vi "sonic info (SubVI).vi"(8 "error in (no error)":errorcluster) -> (0 "error out":errorcluster, 3 "distance to the side":u32)   [LabVIEW 2017]
uses:
  <vilib>/Instr/_visa.llb/VISA Configure Serial Port (Instr).vi
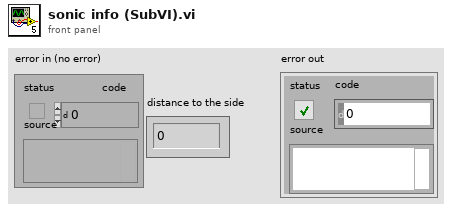
[diagram p1: front panel]
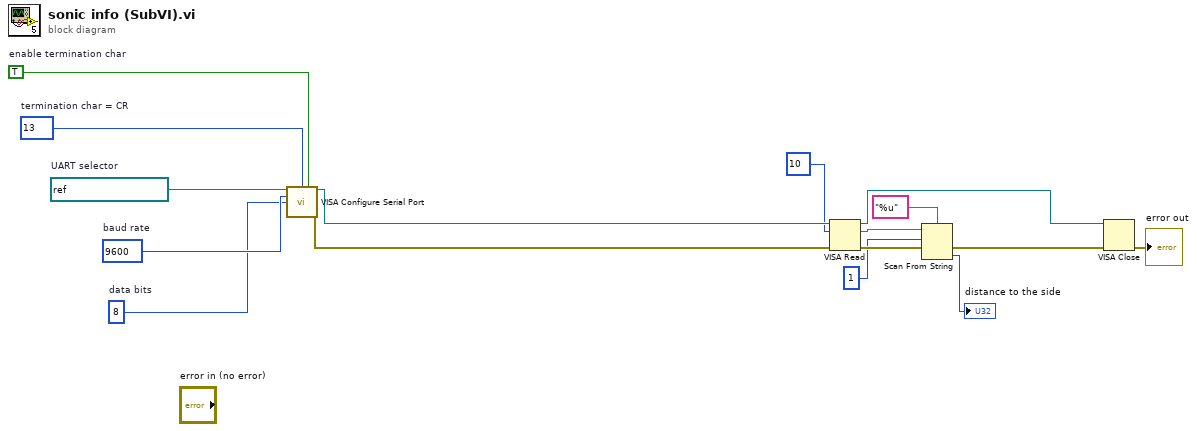
[diagram p0: block diagram]
diagram:
  w12 = u8 13  # termination char = CR
  w13 = refnum<visa-resource-name> "ASRL2::INSTR"  # UART selector
  w11 = TRUE  # enable termination char
  w9 = u16 8  # data bits
  w10 = u32 9600  # baud rate
  n1 = call-poly "VISA Configure Serial Port"("VISA resource name"=w13, "termination char\n(0xA = '\\n' = LF)"=w12, "Enable Termination\nChar (T)"=w11, "baud rate (9600)"=w10, "data bits (8)"=w9) -> ("VISA resource name out"=w8:refnum<visa-resource-name>, "error out"=w7:errorcluster)  [unwired: 9 in]
  n2 = VISA Read(VISA resource name=w8, byte count=u32 10, error in (no error)=w7) -> (VISA resource name out=w14:refnum<visa-resource-name>, read buffer=w4:string, error out=w5:errorcluster)  [unwired: 1 out]
  n3 = Scan From String(format string="%u", input string=w4, initial scan location=u32 1, error in=w5) -> (error out=w16:errorcluster, output 1=→"distance to the side":u32)  [unwired: 1 in, 2 out]
  n4 = VISA Close(VISA resource name=w14, error in (no error)=w16) -> (error out=→"error out":errorcluster)
